vi "Destroy.vi"(8 "error in (no error)":errorcluster, 11 "EventDaemon in":refnum<class "TemplateDaemon.lvclass">) -> (0 "error out":errorcluster)   [LabVIEW 2020, in "TemplateDaemon.lvclass"]
doc: "Destroys events and queues of deamon"
uses:
  TemplateDaemon.lvclass
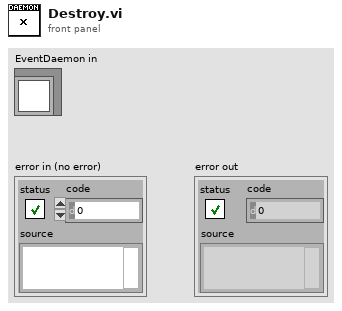
[diagram p1: front panel]
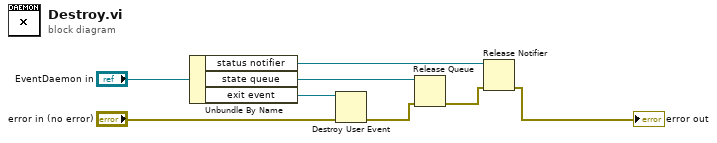
[diagram p0: block diagram]
diagram:
  n1 = Unbundle By Name("EventDaemon in") -> ("status notifier"=w3:refnum<notifier>, "state queue"=w5:refnum<queue>, "exit event"=w7:refnum<user-event>)
  n2 = Destroy User Event(user event=w7, error in="error in (no error)") -> (error out=w4:errorcluster)
  n3 = Release Queue(queue=w5, error in (no error)=w4) -> (error out=w2:errorcluster)  [unwired: 1 in, 2 out]
  n4 = Release Notifier(notifier=w3, error in (no error)=w2) -> (error out=→"error out":errorcluster)  [unwired: 1 in, 2 out]
